vi "Swerve Drive 2020.vi"() -> ()   [LabVIEW 2018]
uses:
  <vilib>/Rock Robotics/WPI/ThirdParty/REV Robotics/SPARK MAX/Typedef/Spark MAX Control Type.ctl
  <vilib>/Rock Robotics/WPI/ThirdParty/Phoenix-LabVIEW/Motor Controller/Controls/CTRE_Phoenix_MotorControl_ControlMode.ctl
  Robot Global Data.vi
  <vilib>/Rock Robotics/WPI/ThirdParty/REV Robotics/SPARK MAX/Typedef/Spark MAX Idle Mode.ctl
  <vilib>/Rock Robotics/WPI/ThirdParty/Phoenix-LabVIEW/Motor Controller/Controls/CTRE_Phoenix_MotorControl_NeutralMode.ctl
panel:
  out "Drive Loop Speed":u32=31
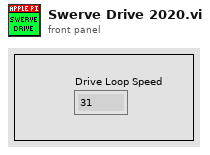
[diagram p1: front panel]
types:
  T1 = enum16{"Sparkmax Brushless", "Talon SRX Brushed"}
  T2 = typedef "WPI_MotorControlDeviceRef.ctl" = cluster{"DeviceStatus":errorcluster, "Type":T3, "PWM":cluster{"PWM Channel":T4, "DeadBand":T5}, "CAN":cluster{"Device Number":u8, "SetOutput VI Ref":variant, "GetOutput VI Ref":variant, "Enable VI Ref":variant, "Disable VI Ref":variant, "Data":variant}, "Invert":bool, "DIO PWM":cluster{"PWM \"Enable\" Channel":T4, "DIOChannel":T6, "PWM Rate":dbl}}
  T3 = typedef "WPI_MotorControlType.ctl" = enum16{"PWM", "CAN", "DIO PWM"}
  T4 = typedef "FPGA_DIOPWMChannel.ctl" = enum8{"PWM 0", "PWM 1", "PWM 2", "PWM 3", "PWM 4", "PWM 5", "PWM 6", "PWM 7", "PWM 8", "PWM 9", "PWM MXP 0", "PWM MXP 1", "PWM MXP 2", "PWM MXP 3", "PWM MXP 4", "PWM MXP 5", "PWM MXP 6", "PWM MXP 7", "PWM MXP 8", "PWM MXP 9", "Invalid"}
  T5 = typedef "WPI_PWMDeadband.ctl" = cluster{"Name":string, "maxPositivePwm":i32, "minPositivePwm":i32, "centerPwm":i32, "maxNegativePwm":i32, "minNegativePwm":i32, "angularRange":u16}
  T6 = typedef "FPGA_DIOChannel.ctl" = enum8{"DIO 0", "DIO 1", "DIO 2", "DIO 3", "DIO 4", "DIO 5", "DIO 6", "DIO 7", "DIO 8", "DIO 9", "DIO MXP 0", "DIO MXP 1", "DIO MXP 2", "DIO MXP 3", "DIO MXP 4", "DIO MXP 5", "DIO MXP 6", "DIO MXP 7", "DIO MXP 8", "DIO MXP 9", "DIO MXP 10", "DIO MXP 11", "DIO MXP 12", "DIO MXP 13", "DIO MXP 14", "DIO MXP 15", "SPI Port CS1", "SPI Port CS2", "SPI Port CS3", "SPI Port MISO", "SPI Port MOSI", "Invalid"}
  T7 = typedef "Spark MAX Control Type.ctl" = enum16{"Percent VBus", "Voltage", "Velocity", "Position"}
  T8 = typedef "CTRE_Phoenix_MotorControl_ControlMode.ctl" = u16
  T9 = typedef "Spark MAX Idle Mode.ctl" = enum16{"Coast", "Brake"}
  T10 = typedef "CTRE_Phoenix_MotorControl_NeutralMode.ctl" = enum8{"EEPROMSetting", "Override to Coast", "Override to Brake"}
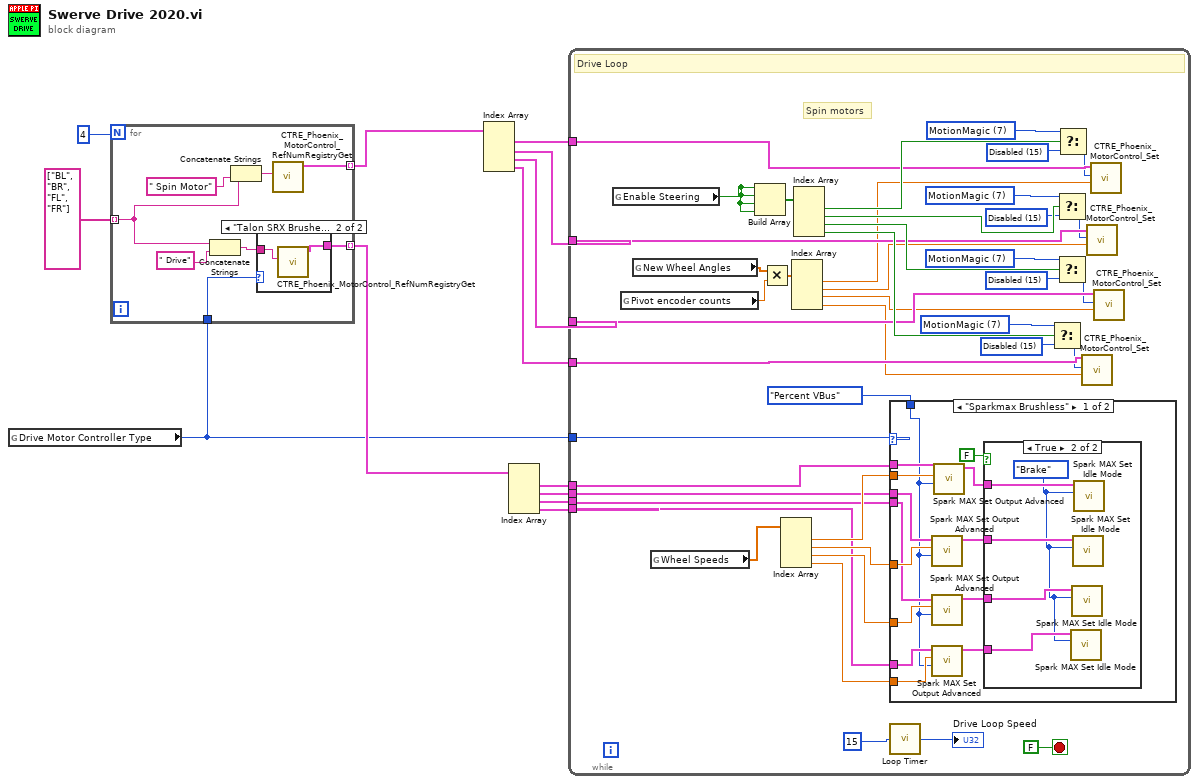
[diagram p0: block diagram]
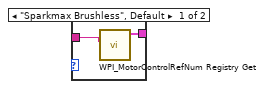
[diagram p2: hidden frame]
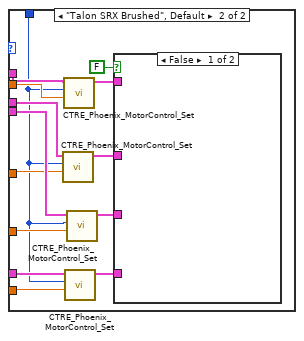
[diagram p4: hidden frame]
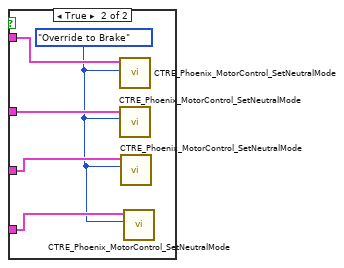
[diagram p5: hidden frame]
diagram:
  n1 = global read "Robot Global Data.vi" "Drive Motor Controller Type"() -> (w1:T1)
  n2 = for {
    N: 4 -> [_]
    tunnel: string[] ["BL", "BR", "FL", "FR"] -> [w21] mode=indexing
    tunnel: [w18] -> w2 mode=indexing
    tunnel: [w16] -> w3 mode=indexing
    tunnel: w1 -> [w14]
    n3 = Concatenate Strings(w21, " Drive") -> (w15:string)
    n4 = Concatenate Strings(w21, " Spin Motor" ("refnum name")) -> (w20:string)
    n5 = case shown="\"Talon SRX Brushed\"" w14 {
      tunnel: [w23 w24] -> w16
      tunnel: w15 -> [w22 w25]
      frame "Sparkmax Brushless", Default {
        n6 = call <vilib>:"WPI_MotorControlRefNum Registry Get.vi"("refnum name"=w22) -> ("MotorControlDevRef"=w23:T2)  [unwired: 9 in, 1 out]
      }
      frame "Talon SRX Brushed" {
        n7 = call <vilib>:"CTRE_Phoenix_MotorControl_RefNumRegistryGet.vi"("refnum name"=w25) -> ("PhoenixMotorControlDevRef"=w24:T2)  [unwired: 9 in, 1 out]
      }
    }
    n8 = call <vilib>:"CTRE_Phoenix_MotorControl_RefNumRegistryGet.vi"("refnum name"=w20) -> ("PhoenixMotorControlDevRef"=w18:T2)  [unwired: 9 in, 1 out]
  }
  n9 = Index Array(array=w2) -> (element #1=w11:T2, element #2=w10:T2, element #3=w4:T2, element #4=w9:T2)  [unwired: 4 in]
  n10 = Index Array(array=w3) -> (element #1=w8:T2, element #2=w7:T2, element #3=w6:T2, element #4=w5:T2)  [unwired: 4 in]
  n11 = while {
    tunnel: w11 -> [w63]
    tunnel: w8 -> [w54]
    tunnel: w10 -> [w62]
    tunnel: w4 -> [w61]
    tunnel: w9 -> [w60]
    tunnel: w7 -> [w53]
    tunnel: w6 -> [w51]
    tunnel: w5 -> [w49]
    tunnel: w1 -> [w29]
    stop <- FALSE stop-if-true
    w36 = T8 15 items=["PercentOutput"=0, "Position"=1, "Velocity"=2, "Current"=3, "Follower"=5, "MotionProfile"=6, "MotionMagic"=7, "MotionMagicArc"=8, "MotionProfileArc"=10, "Disabled"=15] ("Control Mode")
    w37 = T8 7 items=["PercentOutput"=0, "Position"=1, "Velocity"=2, "Current"=3, "Follower"=5, "MotionProfile"=6, "MotionMagic"=7, "MotionMagicArc"=8, "MotionProfileArc"=10, "Disabled"=15] ("Control Mode")
    w38 = T8 15 items=["PercentOutput"=0, "Position"=1, "Velocity"=2, "Current"=3, "Follower"=5, "MotionProfile"=6, "MotionMagic"=7, "MotionMagicArc"=8, "MotionProfileArc"=10, "Disabled"=15] ("Control Mode")
    w39 = T8 7 items=["PercentOutput"=0, "Position"=1, "Velocity"=2, "Current"=3, "Follower"=5, "MotionProfile"=6, "MotionMagic"=7, "MotionMagicArc"=8, "MotionProfileArc"=10, "Disabled"=15] ("Control Mode")
    w42 = T8 15 items=["PercentOutput"=0, "Position"=1, "Velocity"=2, "Current"=3, "Follower"=5, "MotionProfile"=6, "MotionMagic"=7, "MotionMagicArc"=8, "MotionProfileArc"=10, "Disabled"=15] ("Control Mode")
    w43 = T8 7 items=["PercentOutput"=0, "Position"=1, "Velocity"=2, "Current"=3, "Follower"=5, "MotionProfile"=6, "MotionMagic"=7, "MotionMagicArc"=8, "MotionProfileArc"=10, "Disabled"=15] ("Control Mode")
    w46 = T8 15 items=["PercentOutput"=0, "Position"=1, "Velocity"=2, "Current"=3, "Follower"=5, "MotionProfile"=6, "MotionMagic"=7, "MotionMagicArc"=8, "MotionProfileArc"=10, "Disabled"=15] ("Control Mode")
    w45 = T8 7 items=["PercentOutput"=0, "Position"=1, "Velocity"=2, "Current"=3, "Follower"=5, "MotionProfile"=6, "MotionMagic"=7, "MotionMagicArc"=8, "MotionProfileArc"=10, "Disabled"=15] ("Control Mode")
    # "Spin motors"
    # "Drive Loop"
    n12 = global read "Robot Global Data.vi" "Enable Steering"() -> (w32:bool)
    n13 = global read "Robot Global Data.vi" "Pivot encoder counts"() -> (w26:dbl)
    n14 = global read "Robot Global Data.vi" "New Wheel Angles"() -> (w34:dbl[])
    n15 = global read "Robot Global Data.vi" "Wheel Speeds"() -> (w30:dbl[])
    n16 = Build Array(w32, w32, w32, w32) -> (w31:bool[])
    n17 = Multiply(x=w34, y=w26) -> (x*y=w33:dbl[])
    n18 = Index Array(array=w30) -> (element #1=w55:dbl, element #2=w52:dbl, element #3=w50:dbl, element #4=w48:dbl)  [unwired: 4 in]
    n19 = Index Array(array=w33) -> (element #1=w59:dbl, element #2=w58:dbl, element #3=w57:dbl, element #4=w56:dbl)  [unwired: 4 in]
    n20 = Index Array(array=w31) -> (element #1=w64:bool, element #2=w67:bool, element #3=w66:bool, element #4=w65:bool)  [unwired: 4 in]
    n21 = case shown="\"Sparkmax Brushless\"" w29 {
      tunnel: w55 -> [w82 w100]
      tunnel: w54 -> [w81 w101]
      tunnel: w53 -> [w80 w99]
      tunnel: w52 -> [w79 w96]
      tunnel: w51 -> [w78 w98]
      tunnel: w50 -> [w77 w95]
      tunnel: w49 -> [w76 w97]
      tunnel: w48 -> [w75 w94]
      tunnel: Spark_MAX_Control_Type."Percent VBus" ("Control Mode") -> [w74 w93]
      frame "Sparkmax Brushless" {
        n22 = call <vilib>:"Spark MAX Set Output Advanced.vi"("Control Mode"=w74, "Setpoint"=w79, "MotorControlDevRef"=w80) -> ("MotorControlDevRef"=w72:T2)  [unwired: 7 in, 1 out]
        n23 = call <vilib>:"Spark MAX Set Output Advanced.vi"("Control Mode"=w74, "Setpoint"=w77, "MotorControlDevRef"=w78) -> ("MotorControlDevRef"=w71:T2)  [unwired: 7 in, 1 out]
        n24 = call <vilib>:"Spark MAX Set Output Advanced.vi"("Control Mode"=w74, "Setpoint"=w75, "MotorControlDevRef"=w76) -> ("MotorControlDevRef"=w70:T2)  [unwired: 7 in, 1 out]
        n25 = call <vilib>:"Spark MAX Set Output Advanced.vi"("Control Mode"=w74, "Setpoint"=w82, "MotorControlDevRef"=w81) -> ("MotorControlDevRef"=w73:T2)  [unwired: 7 in, 1 out]
        n26 = case shown="True" FALSE {
          tunnel: w73 -> [_ w87]
          tunnel: w72 -> [_ w86]
          tunnel: w71 -> [_ w85]
          tunnel: w70 -> [_ w84]
          frame False {
          }
          frame True {
            w83 = Spark_MAX_Idle_Mode."Brake" ("Idle Mode")
            n27 = call <vilib>:"Spark MAX Set Idle Mode.vi"("Idle Mode"=w83, "MotorControlDeviceRef in"=w84) -> ()  [unwired: 8 in, 2 out]
            n28 = call <vilib>:"Spark MAX Set Idle Mode.vi"("Idle Mode"=w83, "MotorControlDeviceRef in"=w85) -> ()  [unwired: 8 in, 2 out]
            n29 = call <vilib>:"Spark MAX Set Idle Mode.vi"("Idle Mode"=w83, "MotorControlDeviceRef in"=w86) -> ()  [unwired: 8 in, 2 out]
            n30 = call <vilib>:"Spark MAX Set Idle Mode.vi"("Idle Mode"=w83, "MotorControlDeviceRef in"=w87) -> ()  [unwired: 8 in, 2 out]
          }
        }
      }
      frame "Talon SRX Brushed", Default {
        n31 = call <vilib>:"CTRE_Phoenix_MotorControl_Set.vi"("Output"=w96, "Control Mode"=w93, "PhoenixMotorControlDevRef"=w99) -> ("PhoenixMotorControlDevRef"=w89:T2)  [unwired: 7 in, 1 out]
        n32 = call <vilib>:"CTRE_Phoenix_MotorControl_Set.vi"("Output"=w100, "Control Mode"=w93, "PhoenixMotorControlDevRef"=w101) -> ("PhoenixMotorControlDevRef"=w92:T2)  [unwired: 7 in, 1 out]
        n33 = call <vilib>:"CTRE_Phoenix_MotorControl_Set.vi"("Output"=w94, "Control Mode"=w93, "PhoenixMotorControlDevRef"=w97) -> ("PhoenixMotorControlDevRef"=w91:T2)  [unwired: 7 in, 1 out]
        n34 = call <vilib>:"CTRE_Phoenix_MotorControl_Set.vi"("Output"=w95, "Control Mode"=w93, "PhoenixMotorControlDevRef"=w98) -> ("PhoenixMotorControlDevRef"=w90:T2)  [unwired: 7 in, 1 out]
        n35 = case shown="False" FALSE {
          tunnel: w92 -> [_ w106]
          tunnel: w91 -> [_ w105]
          tunnel: w90 -> [_ w104]
          tunnel: w89 -> [_ w103]
          frame False {
          }
          frame True {
            w102 = CTRE_Phoenix_MotorControl_NeutralMode."Override to Brake" ("Motor Control Neutral Mode")
            n36 = call <vilib>:"CTRE_Phoenix_MotorControl_SetNeutralMode.vi"("Motor Control Neutral Mode"=w102, "PhoenixMotorControlDevRef"=w106) -> ()  [unwired: 8 in, 2 out]
            n37 = call <vilib>:"CTRE_Phoenix_MotorControl_SetNeutralMode.vi"("Motor Control Neutral Mode"=w102, "PhoenixMotorControlDevRef"=w103) -> ()  [unwired: 8 in, 2 out]
            n38 = call <vilib>:"CTRE_Phoenix_MotorControl_SetNeutralMode.vi"("Motor Control Neutral Mode"=w102, "PhoenixMotorControlDevRef"=w104) -> ()  [unwired: 8 in, 2 out]
            n39 = call <vilib>:"CTRE_Phoenix_MotorControl_SetNeutralMode.vi"("Motor Control Neutral Mode"=w102, "PhoenixMotorControlDevRef"=w105) -> ()  [unwired: 8 in, 2 out]
          }
        }
      }
    }
    n40 = call "Loop Timer.vi"("Wait time"=u32 15 ("millisecond multiple")) -> ("Loop Time"=→"Drive Loop Speed":u32)
    n41 = Select(t=w39, s=w65, f=w38) -> (s? t:f=w40:T8)
    n42 = Select(t=w45, s=w67, f=w46) -> (s? t:f=w44:T8)
    n43 = Select(t=w43, s=w66, f=w42) -> (s? t:f=w41:T8)
    n44 = Select(t=w37, s=w64, f=w36) -> (s? t:f=w35:T8)
    n45 = call <vilib>:"CTRE_Phoenix_MotorControl_Set.vi"("Output"=w56, "Control Mode"=w40, "PhoenixMotorControlDevRef"=w60) -> ()  [unwired: 7 in, 2 out]
    n46 = call <vilib>:"CTRE_Phoenix_MotorControl_Set.vi"("Output"=w58, "Control Mode"=w44, "PhoenixMotorControlDevRef"=w62) -> ()  [unwired: 7 in, 2 out]
    n47 = call <vilib>:"CTRE_Phoenix_MotorControl_Set.vi"("Output"=w59, "Control Mode"=w35, "PhoenixMotorControlDevRef"=w63) -> ()  [unwired: 7 in, 2 out]
    n48 = call <vilib>:"CTRE_Phoenix_MotorControl_Set.vi"("Output"=w57, "Control Mode"=w41, "PhoenixMotorControlDevRef"=w61) -> ()  [unwired: 7 in, 2 out]
  }
